vi "matrix multiplication.vi"() -> ()   [LabVIEW 2020]
panel:
  out "AxB":fxp<+/-,64,32>[](array[numeric])
  in  "B":fxp<+/-,64,32>[](array[numeric])=[0.0, 0.0, 0.0, 0.0, 0.0, 0.0, 0.0, 0.0, 0.0, 0.0, 0.0, 0.0, 0.0, 0.0, 0.0, 0.0]
  in  "A":fxp<+/-,64,32>[](array[numeric])=[0.0, 0.0, 0.0, 0.0, 0.0, 0.0, 0.0, 0.0, 0.0, 0.0, 0.0, 0.0, 0.0, 0.0, 0.0, 0.0]
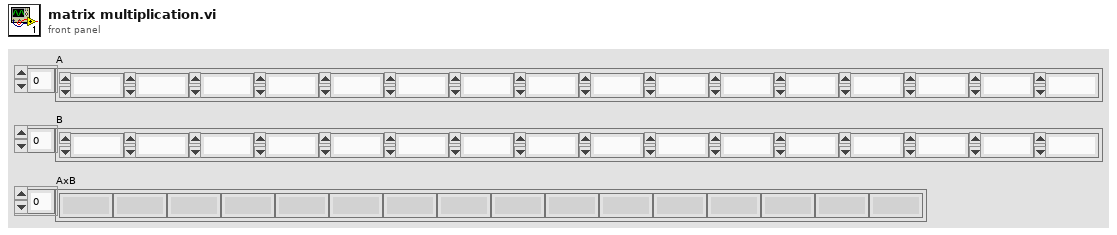
[diagram p1: front panel]
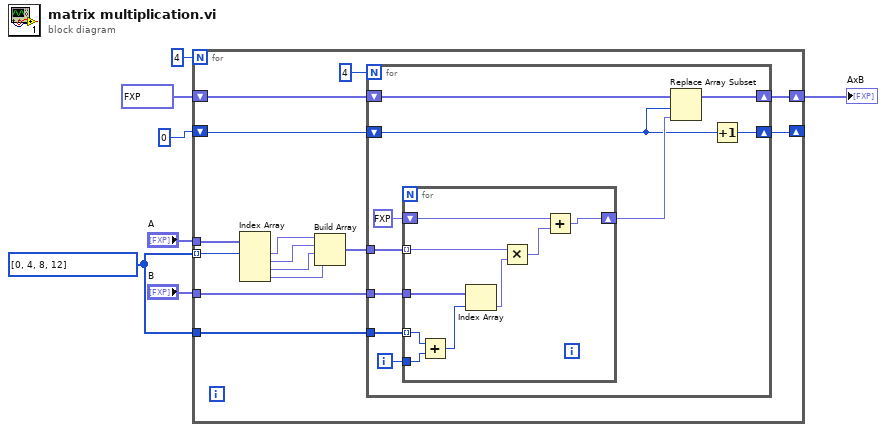
[diagram p0: block diagram]
diagram:
  w6 = i32[] [0, 4, 8, 12]
  n1 = for {
    N: 4 -> [_]
    tunnel: "A" -> [w21]
    tunnel: "B" -> [w20]
    tunnel: w6 -> [w19]
    tunnel: w6 -> [w16] mode=indexing
    shift-right: [w14] -> w1
    shift-left: fxp<+/-,64,32>[] [0.0, 0.0, 0.0, 1.0, 0.0, 0.0, 0.0, 0.0, 0.0, 0.0, 0.0, 0.0, 0.0, 0.0, 0.0, 0.0] ("Appended 1d array 2") -> [w15]
    shift-right: [w12] -> _
    shift-left: 0 ("index") -> [w13]
    n2 = Index Array(array=w21, index #1=w16) -> (element #1=w11:fxp<+/-,64,32>, element #2=w10:fxp<+/-,64,32>, element #3=w9:fxp<+/-,64,32>, element #4=w8:fxp<+/-,64,32>)  [unwired: 3 in]
    n3 = Build Array(w11, w10, w9, w8) -> (w17:fxp<+/-,64,32>[])
    n4 = for {
      N: 4 ("length") -> [_]
      tunnel: w17 -> [w31]
      tunnel: w20 -> [w27]
      tunnel: w19 -> [w29]
      shift-right: [w25] -> w14
      shift-left: w15 -> [w26]
      shift-right: [w22] -> w12
      shift-left: w13 -> [w23]
      i -> [w28]
      n5 = for {
        tunnel: w31 -> [w40] mode=indexing
        shift-right: [w32] -> w24
        shift-left: fxp<+/-,48,32> 0.0 -> [w38]
        tunnel: w29 -> [w37] mode=indexing
        tunnel: w28 -> [w36]
        tunnel: w27 -> [w34]
        n6 = Add(x=w37, y=w36) -> (x+y=w35:i32)
        n7 = Index Array(array=w34, index=w35) -> (element=w33:fxp<+/-,64,32>)
        n8 = Multiply(x=w40, y=w33) -> (x*y=w39:fxp<+/-,48,32>)
        n9 = Add(x=w38, y=w39) -> (x+y=w32:fxp<+/-,48,32>)
      }
      n10 = Replace Array Subset(array=w26, new element=w24, index=w23) -> (w25:fxp<+/-,64,32>[])
      n11 = Increment(x=w23) -> (x+1=w22:i32)
    }
  }
  "AxB" <- w1
